vi "GetBodyParameters.vi"(11 "Parameters":T1[](array[typedef])) -> (2 "HasBodyParameters":bool, 3 "BodyParameters":T1[](array[typedef]))   [LabVIEW 2017, in "MessageGen.lvlib"]
uses:
  <vilib>/addons/InsightCM/MessageBus/CodeGen/MessageGen.lvlib
  <vilib>/addons/InsightCM/MessageBus/CodeGen/controls/Parameter.ctl
  <vilib>/addons/InsightCM/MessageBus/CodeGen/controls/ParameterType.ctl
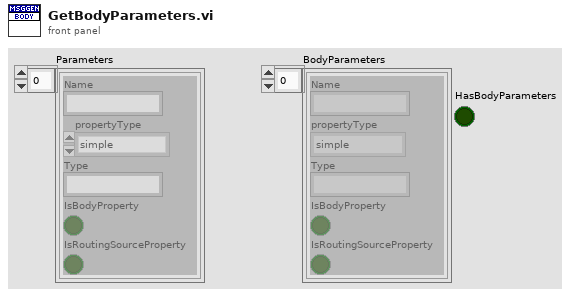
[diagram p1: front panel]
types:
  T1 = typedef "MessageGen.lvlib/Parameter.ctl" = cluster{"Name":string, "propertyType":T2, "Type":string, "IsBodyProperty":bool, "IsRoutingSourceProperty":bool}
  T2 = typedef "MessageGen.lvlib/ParameterType.ctl" = enum16{"simple", "bytearray", "dateTime", "list", "map", "object"}
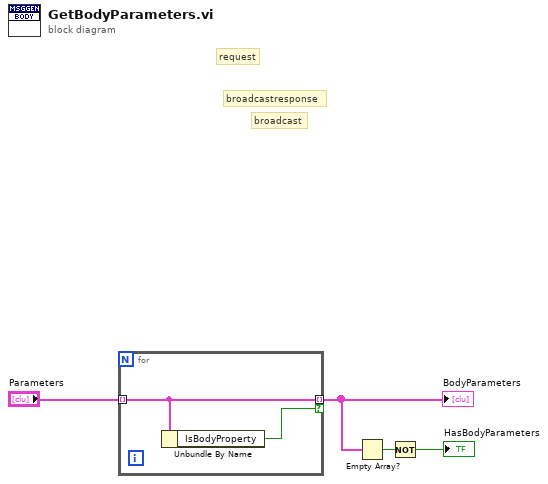
[diagram p0: block diagram]
diagram:
  # "broadcast"
  # "broadcastresponse"
  # "request"
  n1 = for {
    tunnel: "Parameters" -> [w6] mode=indexing
    tunnel: [w6] -> w2 mode=indexing if=w5
    n2 = Unbundle By Name(w6) -> ("IsBodyProperty"=w5:bool)
  }
  "BodyParameters" <- w2
  n3 = Empty Array?(array=w2) -> (empty?=w3:bool)
  n4 = Not(x=w3) -> (.not. x?=→"HasBodyParameters":bool)
